vi "Logger.Variant.FindData4.vi"() -> ()   [LabVIEW 2016] (continued)
"976000107050008691717", "976000107050008701717", "976000107050008711717", "976000107050008721717", "976000107050008731717", "976000107050008741717", "976000107050008751717", "976000107050008761717", "976000107050008771717", "976000107050008781717", "976000107050008791717", "976000107050008801717", "976000107050008811717", "976000107050008821717", "976000107050008831717", "976000107050008841717", "976000107050008851717", "976000107050008861717", "976000107050008871717", "976000107050008881717", "976000107050008891717", "976000107050008901717", "976000107050008911717", "976000107050008921717", "976000107050008931717", "976000107050008941717", "976000107050008951717", "976000107050008961717", "976000107050008971717", "976000107050008981717", "976000107050008991717", "976000107050009001717", "976000107050009011717", "976000107050009021717", "976000107050009031717", "976000107050009041717", "976000107050009051717", "976000107050009061717", "976000107050009071717", "976000107050009081717", "976000107050009091717", "976000107050009101717", "976000107050009111717", "976000107050009121717", "976000107050009131717", "976000107050009141717", "976000107050009151717", "976000107050009161717", "976000107050009171717", "976000107050009181717", "976000107050009191717", "976000107050009201717", "976000107050009211717", "976000107050009221717", "976000107050009231717", "976000107050009241717", "976000107050009251717", "976000107050009261717", "976000107050009271717", "976000107050009281717", "976000107050009291717", "976000107050009301717", "976000107050009311717", "976000107050009321717", "976000107050009331717", "976000107050009341717", "976000107050009351717", "976000107050009361717", "976000107050009371717", "976000107050009381717", "976000107050009391717", "976000107050009401717", "976000107050009411717", "976000107050009421717", "976000107050009431717", "976000107050009441717", "976000107050009451717", "976000107050009461717", "976000107050009471717", "976000107050009481717", "976000107050009491717", "976000107050009501717", "976000107050009511717", "976000107050009521717", "976000107050009531717", "976000107050009541717", "976000107050009551717", "976000107050009561717", "976000107050009571717", "976000107050009581717", "976000107050009591717", "976000107050009601717", "976000107050009611717", "976000107050009621717", "976000107050009631717", "976000107050009641717", "976000107050009651717", "976000107050009661717", "976000107050009671717", "976000107050009681717", "976000107050009691717", "976000107050009701717", "976000107050009711717", "976000107050009721717", "976000107050009731717", "976000107050009741717", "976000107050009751717", "976000107050009761717", "976000107050009771717", "976000107050009781717", "976000107050009791717", "976000107050009801717", "976000107050009811717", "976000107050009821717"]}, {"Product"="4802040310", "Plate"="8990538144", "Path"=path "D:/Maszup/WABCO/SVN/LaserMarkingStation/SOFTWARE/logs/results2/new/170426104556 899 053 814 4.tdms", "Serials"=["480204031053243421717", "480204031053243431717", "480204031053243441717", "480204031053243451717", "480204031053243461717", "480204031053243471717", "480204031053243481717", "480204031053243491717", "480204031053243501717", "480204031053243511717", "480204031053243521717", "480204031053243531717", "480204031053243541717", "480204031053243551717", "480204031053243561717", "480204031053243571717", "480204031053243581717", "480204031053243591717", "480204031053243601717", "480204031053243611717", "480204031053243621717", "480204031053243631717", "480204031053243641717", "480204031053243651717", "480204031053243661717", "480204031053243671717", "480204031053243681717", "480204031053243691717", "480204031053243701717", "480204031053243711717", "480204031053243721717", "480204031053243731717", "480204031053243741717", "480204031053243751717", "480204031053243761717", "480204031053243771717", "480204031053243781717", "480204031053243791717", "480204031053243801717", "480204031053243811717", "480204031053243821717", "480204031053243831717", "480204031053243841717", "480204031053243851717", "480204031053243861717"]}, {"Product"="4728900600", "Plate"="8990538144", "Path"=path "D:/Maszup/WABCO/SVN/LaserMarkingStation/SOFTWARE/logs/results2/new/170426104959 899 053 814 4.tdms", "Serials"=["472890060053240011717", "472890060053240021717", "472890060053240031717", "472890060053240041717", "472890060053240051717", "472890060053240061717", "472890060053240071717", "472890060053240081717", "472890060053240091717", "472890060053240101717", "472890060053240111717", "472890060053240121717", "472890060053240131717", "472890060053240141717", "472890060053240151717", "472890060053240161717", "472890060053240171717", "472890060053240181717", "472890060053240191717", "472890060053240201717", "472890060053240211717", "472890060053240221717", "472890060053240231717", "472890060053240241717"]}, {"Product"="4728900600", "Plate"="8990538144", "Path"=path "D:/Maszup/WABCO/SVN/LaserMarkingStation/SOFTWARE/logs/results2/new/170426105319 899 053 814 4.tdms", "Serials"=["472890060053240251717", "472890060053240261717", "472890060053240271717", "472890060053240281717", "472890060053240291717", "472890060053240301717", "472890060053240311717", "472890060053240321717", "472890060053240331717", "472890060053240341717", "472890060053240351717", "472890060053240361717", "472890060053240371717", "472890060053240381717", "472890060053240391717", "472890060053240401717", "472890060053240411717", "472890060053240421717", "472890060053240431717", "472890060053240441717", "472890060053240451717", "472890060053240461717", "472890060053240471717", "472890060053240481717"]}, {"Product"="4801020650", "Plate"="8990538034", "Path"=path "D:/Maszup/WABCO/SVN/LaserMarkingStation/SOFTWARE/logs/results2/new/170426105704 899 053 803 4.tdms", "Serials"=["48010206500635291717", "48010206500635301717", "48010206500635311717", "48010206500635321717", "48010206500635331717", "48010206500635341717", "48010206500635351717", "48010206500635361717", "48010206500635371717", "48010206500635381717", "48010206500635391717", "48010206500635401717", "48010206500635411717", "48010206500635421717", "48010206500635431717", "48010206500635441717", "48010206500635451717", "48010206500635461717", "48010206500635471717", "48010206500635481717", "48010206500635491717", "48010206500635501717", "48010206500635511717", "48010206500635521717", "48010206500635531717", "48010206500635541717", "48010206500635551717", "48010206500635561717", "48010206500635571717", "48010206500635581717", "48010206500635591717", "48010206500635601717", "48010206500635611717", "48010206500635621717", "48010206500635631717", "48010206500635641717"]}, {"Product"="4801020650", "Plate"="8990538034", "Path"=path "D:/Maszup/WABCO/SVN/LaserMarkingStation/SOFTWARE/logs/results2/new/170426110126 899 053 803 4.tdms", "Serials"=["48010206500634931717", "48010206500634941717", "48010206500634951717", "48010206500634961717", "48010206500634971717", "48010206500634981717", "48010206500634991717", "48010206500635001717", "48010206500635011717", "48010206500635021717", "48010206500635031717", "48010206500635041717", "48010206500635051717", "48010206500635061717", "48010206500635071717", "48010206500635081717", "48010206500635091717", "48010206500635101717", "48010206500635111717", "48010206500635121717", "48010206500635131717", "48010206500635141717", "48010206500635151717", "48010206500635161717", "48010206500635171717", "48010206500635181717", "48010206500635191717", "48010206500635201717", "48010206500635211717", "48010206500635221717", "48010206500635231717", "48010206500635241717", "48010206500635251717", "48010206500635261717", "48010206500635271717", "48010206500635281717"]}, {"Product"="4801020630", "Plate"="8990538034", "Path"=path "D:/Maszup/WABCO/SVN/LaserMarkingStation/SOFTWARE/logs/results2/new/170426110834 899 053 803 4.tdms", "Serials"=["48010206303717401717", "48010206303717411717"]}, {"Product"="4801020630", "Plate"="8990538034", "Path"=path "D:/Maszup/WABCO/SVN/LaserMarkingStation/SOFTWARE/logs/results2/new/170426111204 899 053 803 4.tdms", "Serials"=["48010206303717401717", "48010206303717411717", "48010206303717421717", "48010206303717431717"]}, {"Product"="4801020630", "Plate"="8990538034", "Path"=path "D:/Maszup/WABCO/SVN/LaserMarkingStation/SOFTWARE/logs/results2/new/170426111329 899 053 803 4.tdms", "Serials"=["48010206303717401717", "48010206303717411717", "48010206303717421717", "48010206303717431717", "48010206303717441717", "48010206303717451717", "48010206303717461717", "48010206303717471717", "48010206303717481717", "48010206303717491717", "48010206303717501717", "48010206303717511717", "48010206303717521717", "48010206303717531717", "48010206303717541717", "48010206303717551717", "48010206303717561717", "48010206303717571717", "48010206303717581717", "48010206303717591717", "48010206303717601717", "48010206303717611717", "48010206303717621717", "48010206303717631717"]}, {"Product"="4801020630", "Plate"="8990538034", "Path"=path "D:/Maszup/WABCO/SVN/LaserMarkingStation/SOFTWARE/logs/results2/new/170426112001 899 053 803 4.tdms", "Serials"=["48010206303715961717", "48010206303715971717", "48010206303715981717", "48010206303715991717", "48010206303716001717", "48010206303716011717", "48010206303716021717", "48010206303716031717", "48010206303716041717", "48010206303716051717", "48010206303716061717", "48010206303716071717", "48010206303716081717", "48010206303716091717", "48010206303716101717", "48010206303716111717", "48010206303716121717", "48010206303716131717", "48010206303716141717", "48010206303716151717", "48010206303716161717", "48010206303716171717", "48010206303716181717", "48010206303716191717", "48010206303716201717", "48010206303716211717", "48010206303716221717", "48010206303716231717", "48010206303716241717", "48010206303716251717", "48010206303716261717", "48010206303716271717", "48010206303716281717", "48010206303716291717", "48010206303716301717", "48010206303716311717", "48010206303716321717", "48010206303716331717", "48010206303716341717", "48010206303716351717", "48010206303716361717", "48010206303716371717", "48010206303716381717", "48010206303716391717", "48010206303716401717", "48010206303716411717", "48010206303716421717", "48010206303716431717", "48010206303716441717", "48010206303716451717", "48010206303716461717", "48010206303716471717", "48010206303716481717", "48010206303716491717", "48010206303716501717", "48010206303716511717", "48010206303716521717", "48010206303716531717", "48010206303716541717", "48010206303716551717", "48010206303716561717", "48010206303716571717", "48010206303716581717", "48010206303716591717", "48010206303716601717", "48010206303716611717", "48010206303716621717", "48010206303716631717", "48010206303716641717", "48010206303716651717", "48010206303716661717", "48010206303716671717", "48010206303716681717", "48010206303716691717", "48010206303716701717", "48010206303716711717", "48010206303716721717", "48010206303716731717", "48010206303716741717", "48010206303716751717", "48010206303716761717", "48010206303716771717", "48010206303716781717", "48010206303716791717", "48010206303716801717", "48010206303716811717", "48010206303716821717", "48010206303716831717", "48010206303716841717", "48010206303716851717", "48010206303716861717", "48010206303716871717", "48010206303716881717", "48010206303716891717", "48010206303716901717", "48010206303716911717", "48010206303716921717", "48010206303716931717", "48010206303716941717", "48010206303716951717", "48010206303716961717", "48010206303716971717", "48010206303716981717", "48010206303716991717", "48010206303717001717", "48010206303717011717", "48010206303717021717", "48010206303717031717", "48010206303717041717", "48010206303717051717", "48010206303717061717", "48010206303717071717", "48010206303717081717", "48010206303717091717", "48010206303717101717", "48010206303717111717", "48010206303717121717", "48010206303717131717", "48010206303717141717", "48010206303717151717", "48010206303717161717", "48010206303717171717", "48010206303717181717", "48010206303717191717", "48010206303717201717", "48010206303717211717", "48010206303717221717", "48010206303717231717", "48010206303717241717", "48010206303717251717", "48010206303717261717", "48010206303717271717", "48010206303717281717", "48010206303717291717", "48010206303717301717", "48010206303717311717", "48010206303717321717", "48010206303717331717", "48010206303717341717", "48010206303717351717", "48010206303717361717", "48010206303717371717", "48010206303717381717", "48010206303717391717"]}, {"Product"="4728901120", "Plate"="8990538144", "Path"=path "D:/Maszup/WABCO/SVN/LaserMarkingStation/SOFTWARE/logs/results2/new/170426113518 899 053 814 4.tdms", "Serials"=["472890112055001041717", "472890112055001051717", "472890112055001061717", "472890112055001071717", "472890112055001081717", "472890112055001091717", "472890112055001101717", "472890112055001111717", "472890112055001121717", "472890112055001131717", "472890112055001141717", "472890112055001151717", "472890112055001161717", "472890112055001171717", "472890112055001181717", "472890112055001191717", "472890112055001201717", "472890112055001211717", "472890112055001221717", "472890112055001231717", "472890112055001241717", "472890112055001251717", "472890112055001261717", "472890112055001271717", "472890112055001281717", "472890112055001291717", "472890112055001301717", "472890112055001311717", "472890112055001321717", "472890112055001331717", "472890112055001341717", "472890112055001351717", "472890112055001361717", "472890112055001371717", "472890112055001381717", "472890112055001391717"]}, {"Product"="4729051110", "Plate"="8990538144", "Path"=path "D:/Maszup/WABCO/SVN/LaserMarkingStation/SOFTWARE/logs/results2/new/170426114140 899 053 814 4.tdms", "Serials"=["472905111065780911717", "472905111065780921717", "472905111065780931717", "472905111065780941717", "472905111065780951717", "472905111065780961717", "472905111065780971717", "472905111065780981717", "472905111065780991717", "472905111065781001717", "472905111065781011717", "472905111065781021717", "472905111065781031717", "472905111065781041717", "472905111065781051717", "472905111065781061717", "472905111065781071717", "472905111065781081717", "472905111065781091717", "472905111065781101717"]}, {"Product"="4800030470", "Plate"="8990538144", "Path"=path "D:/Maszup/WABCO/SVN/LaserMarkingStation/SOFTWARE/logs/results2/new/170426115616 899 053 814 4.tdms", "Serials"=["480003047053240031717", "480003047053240041717", "480003047053240051717", "480003047053240061717", "480003047053240071717", "480003047053240081717", "480003047053240091717", "480003047053240101717", "480003047053240111717", "480003047053240121717", "480003047053240131717", "480003047053240141717", "480003047053240151717", "480003047053240161717", "480003047053240171717", "480003047053240181717", "480003047053240191717", "480003047053240201717", "480003047053240211717", "480003047053240221717", "480003047053240231717", "480003047053240241717", "480003047053240251717", "480003047053240261717", "480003047053240271717", "480003047053240281717", "480003047053240291717", "480003047053240301717", "480003047053240311717", "480003047053240321717", "480003047053240331717", "480003047053240341717", "480003047053240351717", "480003047053240361717", "480003047053240371717", "480003047053240381717", "480003047053240391717", "480003047053240401717", "480003047053240411717", "480003047053240421717"]}, {"Product"="4640061000", "Plate"="8990538034", "Path"=path "D:/Maszup/WABCO/SVN/LaserMarkingStation/SOFTWARE/logs/results2/new/170426120944 899 053 803 4.tdms", "Serials"=["46400610000312521717", "46400610000312531717"]}, {"Product"="4800030470", "Plate"="8990538144", "Path"=path "D:/Maszup/WABCO/SVN/LaserMarkingStation/SOFTWARE/logs/results2/new/170426121217 899 053 814 4.tdms", "Serials"=["480003047053240431717", "480003047053240441717", "480003047053240451717", "480003047053240461717", "480003047053240471717", "480003047053240481717", "480003047053240491717", "480003047053240501717", "480003047053240511717", "480003047053240521717", "480003047053240531717", "480003047053240541717", "480003047053240551717", "480003047053240561717", "480003047053240571717", "480003047053240581717", "480003047053240591717", "480003047053240601717", "480003047053240611717", "480003047053240621717", "480003047053240631717", "480003047053240641717", "480003047053240651717", "480003047053240661717", "480003047053240671717", "480003047053240681717", "480003047053240691717", "480003047053240701717", "480003047053240711717", "480003047053240721717", "480003047053240731717", "480003047053240741717", "480003047053240751717", "480003047053240761717", "480003047053240771717", "480003047053240781717", "480003047053240791717", "480003047053240801717", "480003047053240811717", "480003047053240821717"]}, {"Product"="9650010530", "Plate"="8990538144", "Path"=path "D:/Maszup/WABCO/SVN/LaserMarkingStation/SOFTWARE/logs/results2/new/170426150118 899 053 814 4.tdms", "Serials"=["965001053000148491717", "965001053000148501717", "965001053000148511717", "965001053000148521717", "965001053000148531717", "965001053000148541717", "965001053000148551717", "965001053000148561717", "965001053000148571717", "965001053000148581717", "965001053000148591717", "965001053000148601717"]}, {"Product"="9650010530", "Plate"="8990538144", "Path"=path "D:/Maszup/WABCO/SVN/LaserMarkingStation/SOFTWARE/logs/results2/new/170426150640 899 053 814 4.tdms", "Serials"=["965001053000148611717", "965001053000148621717", "965001053000148631717", "965001053000148641717", "965001053000148651717", "965001053000148661717", "965001053000148671717", "965001053000148681717", "965001053000148691717", "965001053000148701717", "965001053000148711717", "965001053000148721717"]}, {"Product"="4800030600", "Plate"="8990501474", "Path"=path "D:/Maszup/WABCO/SVN/LaserMarkingStation/SOFTWARE/logs/results2/new/170426181430 899 050 147 4.tdms", "Serials"=["480003060053240011717", "480003060053240021717", "480003060053240031717", "480003060053240041717", "480003060053240051717", "480003060053240061717", "480003060053240071717", "480003060053240081717", "480003060053240091717", "480003060053240101717", "480003060053240111717", "480003060053240121717", "480003060053240131717", "480003060053240141717", "480003060053240151717", "480003060053240161717", "480003060053240171717", "480003060053240181717", "480003060053240191717", "480003060053240201717", "480003060053240211717", "480003060053240221717", "480003060053240231717", "480003060053240241717"]}, {"Product"="4800030600", "Plate"="8990501474", "Path"=path "D:/Maszup/WABCO/SVN/LaserMarkingStation/SOFTWARE/logs/results2/new/170426181931 899 050 147 4.tdms", "Serials"=["480003060053240251717", "480003060053240261717", "480003060053240271717", "480003060053240281717", "480003060053240291717", "480003060053240301717", "480003060053240311717", "480003060053240321717", "480003060053240331717", "480003060053240341717", "480003060053240351717", "480003060053240361717", "480003060053240371717", "480003060053240381717", "480003060053240391717", "480003060053240401717", "480003060053240411717", "480003060053240421717", "480003060053240431717", "480003060053240441717", "480003060053240451717", "480003060053240461717", "480003060053240471717", "480003060053240481717"]}, {"Product"="4800030500", "Plate"="8990501474", "Path"=path "D:/Maszup/WABCO/SVN/LaserMarkingStation/SOFTWARE/logs/results2/new/170426215055 899 050 147 4.tdms", "Serials"=["480003050053255101717", "480003050053255111717", "480003050053255121717", "480003050053255131717", "480003050053255141717", "480003050053255151717", "480003050053255161717", "480003050053255171717", "480003050053255181717", "480003050053255191717", "480003050053255201717", "480003050053255211717", "480003050053255221717", "480003050053255231717", "480003050053255241717", "480003050053255251717", "480003050053255261717", "480003050053255271717", "480003050053255281717", "480003050053255291717", "480003050053255301717", "480003050053255311717", "480003050053255321717", "480003050053255331717", "480003050053255341717", "480003050053255351717", "480003050053255361717", "480003050053255371717", "480003050053255381717", "480003050053255391717", "480003050053255401717", "480003050053255411717", "480003050053255421717", "480003050053255431717", "480003050053255441717", "480003050053255451717", "480003050053255461717", "480003050053255471717", "480003050053255481717", "480003050053255491717", "480003050053255501717", "480003050053255511717", "480003050053255521717", "480003050053255531717", "480003050053255541717", "480003050053255551717", "480003050053255561717", "480003050053255571717", "480003050053255581717", "480003050053255591717", "480003050053255601717", "480003050053255611717", "480003050053255621717", "480003050053255631717", "480003050053255641717", "480003050053255651717", "480003050053255661717", "480003050053255671717", "480003050053255681717", "480003050053255691717", "480003050053255701717", "480003050053255711717", "480003050053255721717", "480003050053255731717", "480003050053255741717", "480003050053255751717", "480003050053255761717", "480003050053255771717", "480003050053255781717", "480003050053255791717", "480003050053255801717", "480003050053255811717", "480003050053255821717", "480003050053255831717", "480003050053255841717", "480003050053255851717", "480003050053255861717", "480003050053255871717", "480003050053255881717", "480003050053255891717", "480003050053255901717", "480003050053255911717", "480003050053255921717", "480003050053255931717", "480003050053255941717", "480003050053255951717", "480003050053255961717", "480003050053255971717", "480003050053255981717", "480003050053255991717", "480003050053256001717", "480003050053256011717", "480003050053256021717", "480003050053256031717", "480003050053256041717", "480003050053256051717", "480003050053256061717", "480003050053256071717", "480003050053256081717", "480003050053256091717", "480003050053256101717", "480003050053256111717", "480003050053256121717", "480003050053256131717", "480003050053256141717", "480003050053256151717", "480003050053256161717", "480003050053256171717", "480003050053256181717", "480003050053256191717", "480003050053256201717", "480003050053256211717", "480003050053256221717", "480003050053256231717", "480003050053256241717", "480003050053256251717", "480003050053256261717", "480003050053256271717", "480003050053256281717", "480003050053256291717", "480003050053256301717", "480003050053256311717", "480003050053256321717", "480003050053256331717", "480003050053256341717", "480003050053256351717", "480003050053256361717", "480003050053256371717", "480003050053256381717", "480003050053256391717", "480003050053256401717", "480003050053256411717", "480003050053256421717", "480003050053256431717", "480003050053256441717", "480003050053256451717", "480003050053256461717", "480003050053256471717", "480003050053256481717", "480003050053256491717", "480003050053256501717", "480003050053256511717", "480003050053256521717", "480003050053256531717", "480003050053256541717", "480003050053256551717", "480003050053256561717", "480003050053256571717", "480003050053256581717", "480003050053256591717", "480003050053256601717", "480003050053256611717", "480003050053256621717", "480003050053256631717", "480003050053256641717", "480003050053256651717", "480003050053256661717", "480003050053256671717", "480003050053256681717", "480003050053256691717", "480003050053256701717", "480003050053256711717", "480003050053256721717", "480003050053256731717", "480003050053256741717", "480003050053256751717", "480003050053256761717", "480003050053256771717", "480003050053256781717", "480003050053256791717", "480003050053256801717", "480003050053256811717", "480003050053256821717", "480003050053256831717", "480003050053256841717", "480003050053256851717", "480003050053256861717", "480003050053256871717", "480003050053256881717", "480003050053256891717", "480003050053256901717", "480003050053256911717", "480003050053256921717", "480003050053256931717", "480003050053256941717", "480003050053256951717", "480003050053256961717", "480003050053256971717", "480003050053256981717", "480003050053256991717", "480003050053257001717", "480003050053257011717"]}, {"Product"="4728800010", "Plate"="8990538154", "Path"=path "D:/Maszup/WABCO/SVN/LaserMarkingStation/SOFTWARE/logs/results2/new/170427002818 899 053 815 4.tdms", "Serials"=["472880001053240011717"]}, {"Product"="9760001010", "Plate"="8990501474", "Path"=path "D:/Maszup/WABCO/SVN/LaserMarkingStation/SOFTWARE/logs/results2/new/170427061903 899 050 147 4.tdms", "Serials"=["976000101050001241717", "976000101050001251717", "976000101050001261717", "976000101050001271717", "976000101050001281717", "976000101050001291717", "976000101050001301717", "976000101050001311717", "976000101050001321717", "976000101050001331717", "976000101050001341717", "976000101050001351717", "976000101050001361717", "976000101050001371717", "976000101050001381717", "976000101050001391717", "976000101050001401717", "976000101050001411717", "976000101050001421717", "976000101050001431717", "976000101050001441717", "976000101050001451717", "976000101050001461717", "976000101050001471717", "976000101050001481717", "976000101050001491717", "976000101050001501717", "976000101050001511717", "976000101050001521717", "976000101050001531717", "976000101050001541717", "976000101050001551717", "976000101050001561717", "976000101050001571717", "976000101050001581717", "976000101050001591717", "976000101050001601717", "976000101050001611717", "976000101050001621717", "976000101050001631717", "976000101050001641717", "976000101050001651717", "976000101050001661717", "976000101050001671717", "976000101050001681717", "976000101050001691717", "976000101050001701717", "976000101050001711717"]}, {"Product"="4640060027", "Plate"="8990502914", "Path"=path "D:/Maszup/WABCO/SVN/LaserMarkingStation/SOFTWARE/logs/results2/new/170427093837 899 050 291 4.tdms", "Serials"=["46400600270139471717", "46400600270139481717", "46400600270139491717", "46400600270139501717", "46400600270139511717", "46400600270139521717", "46400600270139531717", "46400600270139541717", "46400600270139551717", "46400600270139561717", "46400600270139571717", "46400600270139581717", "46400600270139591717", "46400600270139601717", "46400600270139611717", "46400600270139621717", "46400600270139631717", "46400600270139641717", "46400600270139651717", "46400600270139661717", "46400600270139671717", "46400600270139681717", "46400600270139691717", "46400600270139701717", "46400600270139711717", "46400600270139721717", "46400600270139731717", "46400600270139741717", "46400600270139751717", "46400600270139761717", "46400600270139771717", "46400600270139781717", "46400600270139791717", "46400600270139801717", "46400600270139811717", "46400600270139821717", "46400600270139831717", "46400600270139841717", "46400600270139851717", "46400600270139861717", "46400600270139871717", "46400600270139881717", "46400600270139891717", "46400600270139901717", "46400600270139911717", "46400600270139921717", "46400600270139931717", "46400600270139941717", "46400600270139951717", "46400600270139961717", "46400600270139971717", "46400600270139981717", "46400600270139991717"]}, {"Product"="8840494120", "Plate"="8990538144", "Path"=path "D:/Maszup/WABCO/SVN/LaserMarkingStation/SOFTWARE/logs/results2/new/170427124622 899 053 814 4.tdms", "Serials"=["884049412000000161717", "884049412000000171717", "884049412000000181717"]}, {"Product"="4800030500", "Plate"="8990501474", "Path"=path "D:/Maszup/WABCO/SVN/LaserMarkingStation/SOFTWARE/logs/results2/new/170427130233 899 050 147 4.tdms", "Serials"=["480003050053257021717", "480003050053257031717", "480003050053257041717", "480003050053257051717", "480003050053257061717", "480003050053257071717", "480003050053257081717", "480003050053257091717", "480003050053257101717", "480003050053257111717", "480003050053257121717", "480003050053257131717", "480003050053257141717", "480003050053257151717", "480003050053257161717", "480003050053257171717", "480003050053257181717", "480003050053257191717", "480003050053257201717", "480003050053257211717", "480003050053257221717", "480003050053257231717", "480003050053257241717", "480003050053257251717", "480003050053257261717", "480003050053257271717", "480003050053257281717", "480003050053257291717", "480003050053257301717", "480003050053257311717", "480003050053257321717", "480003050053257331717", "480003050053257341717", "480003050053257351717", "480003050053257361717", "480003050053257371717", "480003050053257381717", "480003050053257391717", "480003050053257401717", "480003050053257411717", "480003050053257421717", "480003050053257431717", "480003050053257441717", "480003050053257451717", "480003050053257461717", "480003050053257471717", "480003050053257481717", "480003050053257491717", "480003050053257501717", "480003050053257511717", "480003050053257521717", "480003050053257531717", "480003050053257541717", "480003050053257551717", "480003050053257561717", "480003050053257571717", "480003050053257581717", "480003050053257591717", "480003050053257601717", "480003050053257611717", "480003050053257621717", "480003050053257631717", "480003050053257641717", "480003050053257651717"]}, {"Product"="4800030500", "Plate"="8990501474", "Path"=path "D:/Maszup/WABCO/SVN/LaserMarkingStation/SOFTWARE/logs/results2/new/170427190006 899 050 147 4.tdms", "Serials"=["480003050053257661717", "480003050053257671717", "480003050053257681717", "480003050053257691717", "480003050053257701717", "480003050053257711717", "480003050053257721717", "480003050053257731717", "480003050053257741717", "480003050053257751717", "480003050053257761717", "480003050053257771717", "480003050053257781717", "480003050053257791717", "480003050053257801717", "480003050053257811717", "480003050053257821717", "480003050053257831717", "480003050053257841717", "480003050053257851717", "480003050053257861717", "480003050053257871717", "480003050053257881717", "480003050053257891717", "480003050053257901717", "480003050053257911717", "480003050053257921717", "480003050053257931717", "480003050053257941717", "480003050053257951717", "480003050053257961717", "480003050053257971717", "480003050053257981717", "480003050053257991717", "480003050053258001717", "480003050053258011717", "480003050053258021717", "480003050053258031717", "480003050053258041717", "480003050053258051717", "480003050053258061717", "480003050053258071717", "480003050053258081717", "480003050053258091717", "480003050053258101717", "480003050053258111717", "480003050053258121717", "480003050053258131717", "480003050053258141717", "480003050053258151717", "480003050053258161717", "480003050053258171717", "480003050053258181717", "480003050053258191717", "480003050053258201717", "480003050053258211717", "480003050053258221717", "480003050053258231717", "480003050053258241717", "480003050053258251717", "480003050053258261717", "480003050053258271717", "480003050053258281717", "480003050053258291717", "480003050053258301717", "480003050053258311717", "480003050053258321717", "480003050053258331717", "480003050053258341717", "480003050053258351717", "480003050053258361717", "480003050053258371717", "480003050053258381717", "480003050053258391717", "480003050053258401717", "480003050053258411717", "480003050053258421717", "480003050053258431717", "480003050053258441717", "480003050053258451717", "480003050053258461717", "480003050053258471717", "480003050053258481717", "480003050053258491717", "480003050053258501717", "480003050053258511717", "480003050053258521717", "480003050053258531717", "480003050053258541717", "480003050053258551717", "480003050053258561717", "480003050053258571717", "480003050053258581717", "480003050053258591717", "480003050053258601717", "480003050053258611717", "480003050053258621717", "480003050053258631717", "480003050053258641717", "480003050053258651717", "480003050053258661717", "480003050053258671717", "480003050053258681717", "480003050053258691717", "480003050053258701717", "480003050053258711717", "480003050053258721717", "480003050053258731717", "480003050053258741717", "480003050053258751717", "480003050053258761717", "480003050053258771717", "480003050053258781717", "480003050053258791717", "480003050053258801717", "480003050053258811717", "480003050053258821717", "480003050053258831717", "480003050053258841717", "480003050053258851717", "480003050053258861717", "480003050053258871717", "480003050053258881717", "480003050053258891717", "480003050053258901717", "480003050053258911717", "480003050053258921717", "480003050053258931717", "480003050053258941717", "480003050053258951717", "480003050053258961717", "480003050053258971717", "480003050053258981717", "480003050053258991717", "480003050053259001717", "480003050053259011717", "480003050053259021717", "480003050053259031717", "480003050053259041717", "480003050053259051717", "480003050053259061717", "480003050053259071717", "480003050053259081717", "480003050053259091717", "480003050053259101717", "480003050053259111717", "480003050053259121717", "480003050053259131717", "480003050053259141717", "480003050053259151717", "480003050053259161717", "480003050053259171717", "480003050053259181717", "480003050053259191717", "480003050053259201717", "480003050053259211717", "480003050053259221717", "480003050053259231717", "480003050053259241717", "480003050053259251717", "480003050053259261717", "480003050053259271717", "480003050053259281717", "480003050053259291717", "480003050053259301717", "480003050053259311717", "480003050053259321717", "480003050053259331717", "480003050053259341717", "480003050053259351717", "480003050053259361717", "480003050053259371717", "480003050053259381717", "480003050053259391717", "480003050053259401717", "480003050053259411717", "480003050053259421717", "480003050053259431717", "480003050053259441717", "480003050053259451717", "480003050053259461717", "480003050053259471717", "480003050053259481717", "480003050053259491717", "480003050053259501717", "480003050053259511717", "480003050053259521717", "480003050053259531717", "480003050053259541717", "480003050053259551717", "480003050053259561717", "480003050053259571717"]}, {"Product"="4800030500", "Plate"="8990501474", "Path"=path "D:/Maszup/WABCO/SVN/LaserMarkingStation/SOFTWARE/logs/results2/new/170427192330 899 050 147 4.tdms", "Serials"=["480003050053259581717", "480003050053259591717", "480003050053259601717", "480003050053259611717", "480003050053259621717", "480003050053259631717", "480003050053259641717", "480003050053259651717", "480003050053259661717", "480003050053259671717", "480003050053259681717", "480003050053259691717", "480003050053259701717", "480003050053259711717", "480003050053259721717", "480003050053259731717", "480003050053259741717", "480003050053259751717", "480003050053259761717", "480003050053259771717", "480003050053259781717", "480003050053259791717", "480003050053259801717", "480003050053259811717", "480003050053259821717", "480003050053259831717", "480003050053259841717", "480003050053259851717", "480003050053259861717", "480003050053259871717", "480003050053259881717", "480003050053259891717", "480003050053259901717", "480003050053259911717", "480003050053259921717", "480003050053259931717", "480003050053259941717", "480003050053259951717", "480003050053259961717", "480003050053259971717", "480003050053259981717", "480003050053259991717", "480003050053260001717", "480003050053260011717", "480003050053260021717", "480003050053260031717", "480003050053260041717", "480003050053260051717", "480003050053260061717", "480003050053260071717", "480003050053260081717", "480003050053260091717", "480003050053260101717", "480003050053260111717", "480003050053260121717", "480003050053260131717", "480003050053260141717", "480003050053260151717", "480003050053260161717", "480003050053260171717", "480003050053260181717", "480003050053260191717", "480003050053260201717", "480003050053260211717", "480003050053260221717", "480003050053260231717", "480003050053260241717", "480003050053260251717", "480003050053260261717", "480003050053260271717", "480003050053260281717", "480003050053260291717", "480003050053260301717", "480003050053260311717", "480003050053260321717", "480003050053260331717", "480003050053260341717", "480003050053260351717", "480003050053260361717", "480003050053260371717", "480003050053260381717", "480003050053260391717", "480003050053260401717", "480003050053260411717", "480003050053260421717", "480003050053260431717", "480003050053260441717", "480003050053260451717", "480003050053260461717", "480003050053260471717", "480003050053260481717", "480003050053260491717", "480003050053260501717", "480003050053260511717", "480003050053260521717", "480003050053260531717", "480003050053260541717", "480003050053260551717", "480003050053260561717", "480003050053260571717", "480003050053260581717", "480003050053260591717", "480003050053260601717", "480003050053260611717", "480003050053260621717", "480003050053260631717", "480003050053260641717", "480003050053260651717", "480003050053260661717", "480003050053260671717", "480003050053260681717", "480003050053260691717", "480003050053260701717", "480003050053260711717", "480003050053260721717", "480003050053260731717", "480003050053260741717", "480003050053260751717", "480003050053260761717", "480003050053260771717", "480003050053260781717", "480003050053260791717", "480003050053260801717", "480003050053260811717", "480003050053260821717", "480003050053260831717", "480003050053260841717", "480003050053260851717", "480003050053260861717", "480003050053260871717", "480003050053260881717", "480003050053260891717", "480003050053260901717", "480003050053260911717", "480003050053260921717", "480003050053260931717", "480003050053260941717", "480003050053260951717", "480003050053260961717", "480003050053260971717", "480003050053260981717", "480003050053260991717", "480003050053261001717", "480003050053261011717", "480003050053261021717", "480003050053261031717", "480003050053261041717", "480003050053261051717", "480003050053261061717", "480003050053261071717", "480003050053261081717", "480003050053261091717", "480003050053261101717", "480003050053261111717", "480003050053261121717", "480003050053261131717", "480003050053261141717", "480003050053261151717", "480003050053261161717", "480003050053261171717", "480003050053261181717", "480003050053261191717", "480003050053261201717", "480003050053261211717", "480003050053261221717", "480003050053261231717", "480003050053261241717", "480003050053261251717", "480003050053261261717", "480003050053261271717", "480003050053261281717", "480003050053261291717", "480003050053261301717", "480003050053261311717", "480003050053261321717", "480003050053261331717", "480003050053261341717", "480003050053261351717", "480003050053261361717", "480003050053261371717", "480003050053261381717", "480003050053261391717", "480003050053261401717", "480003050053261411717", "480003050053261421717", "480003050053261431717", "480003050053261441717", "480003050053261451717", "480003050053261461717", "480003050053261471717", "480003050053261481717", "480003050053261491717"]}, {"Product"="9760001070", "Plate"="8990538144", "Path"=path "D:/Maszup/WABCO/SVN/LaserMarkingStation/SOFTWARE/logs/results2/new/170427233224 899 053 814 4.tdms", "Serials"=["976000107050009831717", "976000107050009841717", "976000107050009851717", "976000107050009861717", "976000107050009871717"]}, {"Product"="9760001010", "Plate"="8990501474", "Path"=path "D:/Maszup/WABCO/SVN/LaserMarkingStation/SOFTWARE/logs/results2/new/170427233422 899 050 147 4.tdms", "Serials"=["976000101050001721717", "976000101050001731717", "976000101050001741717", "976000101050001751717", "976000101050001761717", "976000101050001771717", "976000101050001781717", "976000101050001791717", "976000101050001801717", "976000101050001811717", "976000101050001821717", "976000101050001831717", "976000101050001841717", "976000101050001851717", "976000101050001861717", "976000101050001871717", "976000101050001881717", "976000101050001891717", "976000101050001901717", "976000101050001911717", "976000101050001921717", "976000101050001931717", "976000101050001941717", "976000101050001951717", "976000101050001961717", "976000101050001971717", "976000101050001981717", "976000101050001991717", "976000101050002001717", "976000101050002011717", "976000101050002021717", "976000101050002031717", "976000101050002041717", "976000101050002051717", "976000101050002061717", "976000101050002071717", "976000101050002081717", "976000101050002091717", "976000101050002101717", "976000101050002111717", "976000101050002121717", "976000101050002131717", "976000101050002141717", "976000101050002151717", "976000101050002161717", "976000101050002171717", "976000101050002181717", "976000101050002191717"]}, {"Product"="9760001000", "Plate"="8990501474", "Path"=path "D:/Maszup/WABCO/SVN/LaserMarkingStation/SOFTWARE/logs/results2/new/170427234049 899 050 147 4.tdms", "Serials"=["976000100050000551717", "976000100050000561717"]}, {"Product"="8840550640", "Plate"="8990538144", "Path"=path "D:/Maszup/WABCO/SVN/LaserMarkingStation/SOFTWARE/logs/results2/new/170428092516 899 053 814 4.tdms", "Serials"=["884055064000000011717", "884055064000000021717", "884055064000000031717", "884055064000000041717", "884055064000000051717", "884055064000000061717", "884055064000000071717", "884055064000000081717", "884055064000000091717", "884055064000000101717", "884055064000000111717", "884055064000000121717", "884055064000000131717", "884055064000000141717", "884055064000000151717", "884055064000000161717"]}, {"Product"="8840475770", "Plate"="8990538144", "Path"=path "D:/Maszup/WABCO/SVN/LaserMarkingStation/SOFTWARE/logs/results2/new/170428111110 899 053 814 4.tdms", "Serials"=["884047577050000011717", "884047577050000021717"]}, {"Product"="8840437270", "Plate"="8990538144", "Path"=path "D:/Maszup/WABCO/SVN/LaserMarkingStation/SOFTWARE/logs/results2/new/170428111301 899 053 814 4.tdms", "Serials"=["884043727050000661717", "884043727050000671717", "884043727050000681717", "884043727050000691717", "884043727050000701717", "884043727050000711717", "884043727050000721717"]}, {"Product"="9650010550", "Plate"="8990538144", "Path"=path "D:/Maszup/WABCO/SVN/LaserMarkingStation/SOFTWARE/logs/results2/new/170428113602 899 053 814 4.tdms", "Serials"=["965001055001230191717", "965001055001230201717", "965001055001230211717", "965001055001230221717", "965001055001230231717", "965001055001230241717", "965001055001230251717", "965001055001230261717", "965001055001230271717", "965001055001230281717", "965001055001230291717", "965001055001230301717"]}, {"Product"="9650010550", "Plate"="8990538144", "Path"=path "D:/Maszup/WABCO/SVN/LaserMarkingStation/SOFTWARE/logs/results2/new/170428113814 899 053 814 4.tdms", "Serials"=["965001055001230311717", "965001055001230321717", "965001055001230331717", "965001055001230341717", "965001055001230351717", "965001055001230361717", "965001055001230371717", "965001055001230381717", "965001055001230391717", "965001055001230401717", "965001055001230411717", "965001055001230421717"]}, {"Product"="9650010550", "Plate"="8990538144", "Path"=path "D:/Maszup/WABCO/SVN/LaserMarkingStation/SOFTWARE/logs/results2/new/170428114248 899 053 814 4.tdms", "Serials"=["965001055001230431717", "965001055001230441717", "965001055001230451717", "965001055001230461717", "965001055001230471717", "965001055001230481717", "965001055001230491717", "965001055001230501717", "965001055001230511717", "965001055001230521717", "965001055001230531717", "965001055001230541717"]}, {"Product"="9650010550", "Plate"="8990538144", "Path"=path "D:/Maszup/WABCO/SVN/LaserMarkingStation/SOFTWARE/logs/results2/new/170428114529 899 053 814 4.tdms", "Serials"=["965001055001230551717", "965001055001230561717", "965001055001230571717", "965001055001230581717", "965001055001230591717", "965001055001230601717", "965001055001230611717", "965001055001230621717", "965001055001230631717", "965001055001230641717", "965001055001230651717", "965001055001230661717"]}, {"Product"="4800030580", "Plate"="8990501474", "Path"=path "D:/Maszup/WABCO/SVN/LaserMarkingStation/SOFTWARE/logs/results2/new/170428152705 899 050 147 4.tdms", "Serials"=["480003058053240671717", "480003058053240681717", "480003058053240691717", "480003058053240701717", "480003058053240711717", "480003058053240721717", "480003058053240731717", "480003058053240741717", "480003058053240751717", "480003058053240761717", "480003058053240771717", "480003058053240781717", "480003058053240791717", "480003058053240801717", "480003058053240811717", "480003058053240821717", "480003058053240831717", "480003058053240841717", "480003058053240851717", "480003058053240861717", "480003058053240871717", "480003058053240881717", "480003058053240891717", "480003058053240901717", "480003058053240911717", "480003058053240921717", "480003058053240931717", "480003058053240941717", "480003058053240951717", "480003058053240961717", "480003058053240971717", "480003058053240981717", "480003058053240991717", "480003058053241001717", "480003058053241011717", "480003058053241021717", "480003058053241031717", "480003058053241041717", "480003058053241051717", "480003058053241061717", "480003058053241071717", "480003058053241081717", "480003058053241091717", "480003058053241101717", "480003058053241111717", "480003058053241121717", "480003058053241131717", "480003058053241141717", "480003058053241151717", "480003058053241161717", "480003058053241171717", "480003058053241181717", "480003058053241191717", "480003058053241201717", "480003058053241211717", "480003058053241221717", "480003058053241231717", "480003058053241241717", "480003058053241251717", "480003058053241261717", "480003058053241271717", "480003058053241281717", "480003058053241291717", "480003058053241301717", "480003058053241311717", "480003058053241321717", "480003058053241331717", "480003058053241341717", "480003058053241351717", "480003058053241361717", "480003058053241371717", "480003058053241381717", "480003058053241391717", "480003058053241401717", "480003058053241411717", "480003058053241421717", "480003058053241431717", "480003058053241441717", "480003058053241451717", "480003058053241461717", "480003058053241471717", "480003058053241481717", "480003058053241491717", "480003058053241501717", "480003058053241511717", "480003058053241521717", "480003058053241531717", "480003058053241541717", "480003058053241551717", "480003058053241561717", "480003058053241571717", "480003058053241581717", "480003058053241591717", "480003058053241601717", "480003058053241611717", "480003058053241621717", "480003058053241631717", "480003058053241641717", "480003058053241651717", "480003058053241661717", "480003058053241671717", "480003058053241681717", "480003058053241691717", "480003058053241701717", "480003058053241711717", "480003058053241721717", "480003058053241731717", "480003058053241741717", "480003058053241751717", "480003058053241761717", "480003058053241771717", "480003058053241781717", "480003058053241791717", "480003058053241801717", "480003058053241811717", "480003058053241821717", "480003058053241831717", "480003058053241841717", "480003058053241851717", "480003058053241861717", "480003058053241871717", "480003058053241881717", "480003058053241891717", "480003058053241901717", "480003058053241911717", "480003058053241921717", "480003058053241931717", "480003058053241941717"]}, {"Product"="9760001000", "Plate"="8990501474", "Path"=path "D:/Maszup/WABCO/SVN/LaserMarkingStation/SOFTWARE/logs/results2/new/170428153838 899 050 147 4.tdms", "Serials"=["976000100050000571717", "976000100050000581717", "976000100050000591717", "976000100050000601717", "976000100050000611717", "976000100050000621717", "976000100050000631717", "976000100050000641717", "976000100050000651717", "976000100050000661717", "976000100050000671717", "976000100050000681717", "976000100050000691717", "976000100050000701717", "976000100050000711717", "976000100050000721717"]}, {"Product"="4800030500", "Plate"="8990501474", "Path"=path "D:/Maszup/WABCO/SVN/LaserMarkingStation/SOFTWARE/logs/results2/new/170428171435 899 050 147 4.tdms", "Serials"=["480003050053261501717", "480003050053261511717", "480003050053261521717", "480003050053261531717", "480003050053261541717", "480003050053261551717", "480003050053261561717", "480003050053261571717", "480003050053261581717", "480003050053261591717", "480003050053261601717", "480003050053261611717", "480003050053261621717", "480003050053261631717", "480003050053261641717", "480003050053261651717", "480003050053261661717", "480003050053261671717", "480003050053261681717", "480003050053261691717", "480003050053261701717", "480003050053261711717", "480003050053261721717", "480003050053261731717", "480003050053261741717", "480003050053261751717", "480003050053261761717", "480003050053261771717", "480003050053261781717", "480003050053261791717", "480003050053261801717", "480003050053261811717", "480003050053261821717", "480003050053261831717", "480003050053261841717", "480003050053261851717", "480003050053261861717", "480003050053261871717", "480003050053261881717", "480003050053261891717", "480003050053261901717", "480003050053261911717", "480003050053261921717", "480003050053261931717", "480003050053261941717", "480003050053261951717", "480003050053261961717", "480003050053261971717", "480003050053261981717", "480003050053261991717", "480003050053262001717", "480003050053262011717"]}, {"Product"="4640060027", "Plate"="8990502914", "Path"=path "D:/Maszup/WABCO/SVN/LaserMarkingStation/SOFTWARE/logs/results2/new/170428180206 899 050 291 4.tdms", "Serials"=["46400600270142401717", "46400600270142411717", "46400600270142421717", "46400600270142431717", "46400600270142441717", "46400600270142451717", "46400600270142461717", "46400600270142471717", "46400600270142481717", "46400600270142491717", "46400600270142501717", "46400600270142511717", "46400600270142521717", "46400600270142531717", "46400600270142541717", "46400600270142551717", "46400600270142561717", "46400600270142571717", "46400600270142581717", "46400600270142591717", "46400600270142601717", "46400600270142611717", "46400600270142621717", "46400600270142631717", "46400600270142641717", "46400600270142651717", "46400600270142661717", "46400600270142671717", "46400600270142681717", "46400600270142691717", "46400600270142701717", "46400600270142711717", "46400600270142721717", "46400600270142731717", "46400600270142741717", "46400600270142751717", "46400600270142761717", "46400600270142771717", "46400600270142781717", "46400600270142791717", "46400600270142801717", "46400600270142811717", "46400600270142821717", "46400600270142831717", "46400600270142841717", "46400600270142851717", "46400600270142861717", "46400600270142871717", "46400600270142881717", "46400600270142891717", "46400600270142901717", "46400600270142911717", "46400600270142921717", "46400600270142931717", "46400600270142941717", "46400600270142951717", "46400600270142961717", "46400600270142971717", "46400600270142981717", "46400600270142991717", "46400600270143001717", "46400600270143011717", "46400600270143021717", "46400600270143031717", "46400600270143041717", "46400600270143051717", "46400600270143061717", "46400600270143071717", "46400600270143081717", "46400600270143091717", "46400600270143101717", "46400600270143111717", "46400600270143121717", "46400600270143131717", "46400600270143141717", "46400600270143151717", "46400600270143161717", "46400600270143171717", "46400600270143181717", "46400600270143191717"]}, {"Product"="4728800010", "Plate"="8990538154", "Path"=path "D:/Maszup/WABCO/SVN/LaserMarkingStation/SOFTWARE/logs/results2/old/170420083829 899 053 815 4.tdms", "Serials"=["472880001050001511617", "472880001050001521617", "472880001050001531617", "472880001050001541617", "472880001050001551617", "472880001050001561617", "472880001050001571617", "472880001050001581617", "472880001050001591617", "472880001050001601617", "472880001050001611617", "472880001050001621617", "472880001050001631617", "472880001050001641617", "472880001050001651617"]}, {"Product"="9762001000", "Plate"="8990538144", "Path"=path "D:/Maszup/WABCO/SVN/LaserMarkingStation/SOFTWARE/logs/results2/old/170420085232 899 053 814 4.tdms", "Serials"=["976200100000003891617", "976200100000003901617", "976200100000003911617", "976200100000003921617", "976200100000003931617", "976200100000003941617", "976200100000003951617", "976200100000003961617"]}]
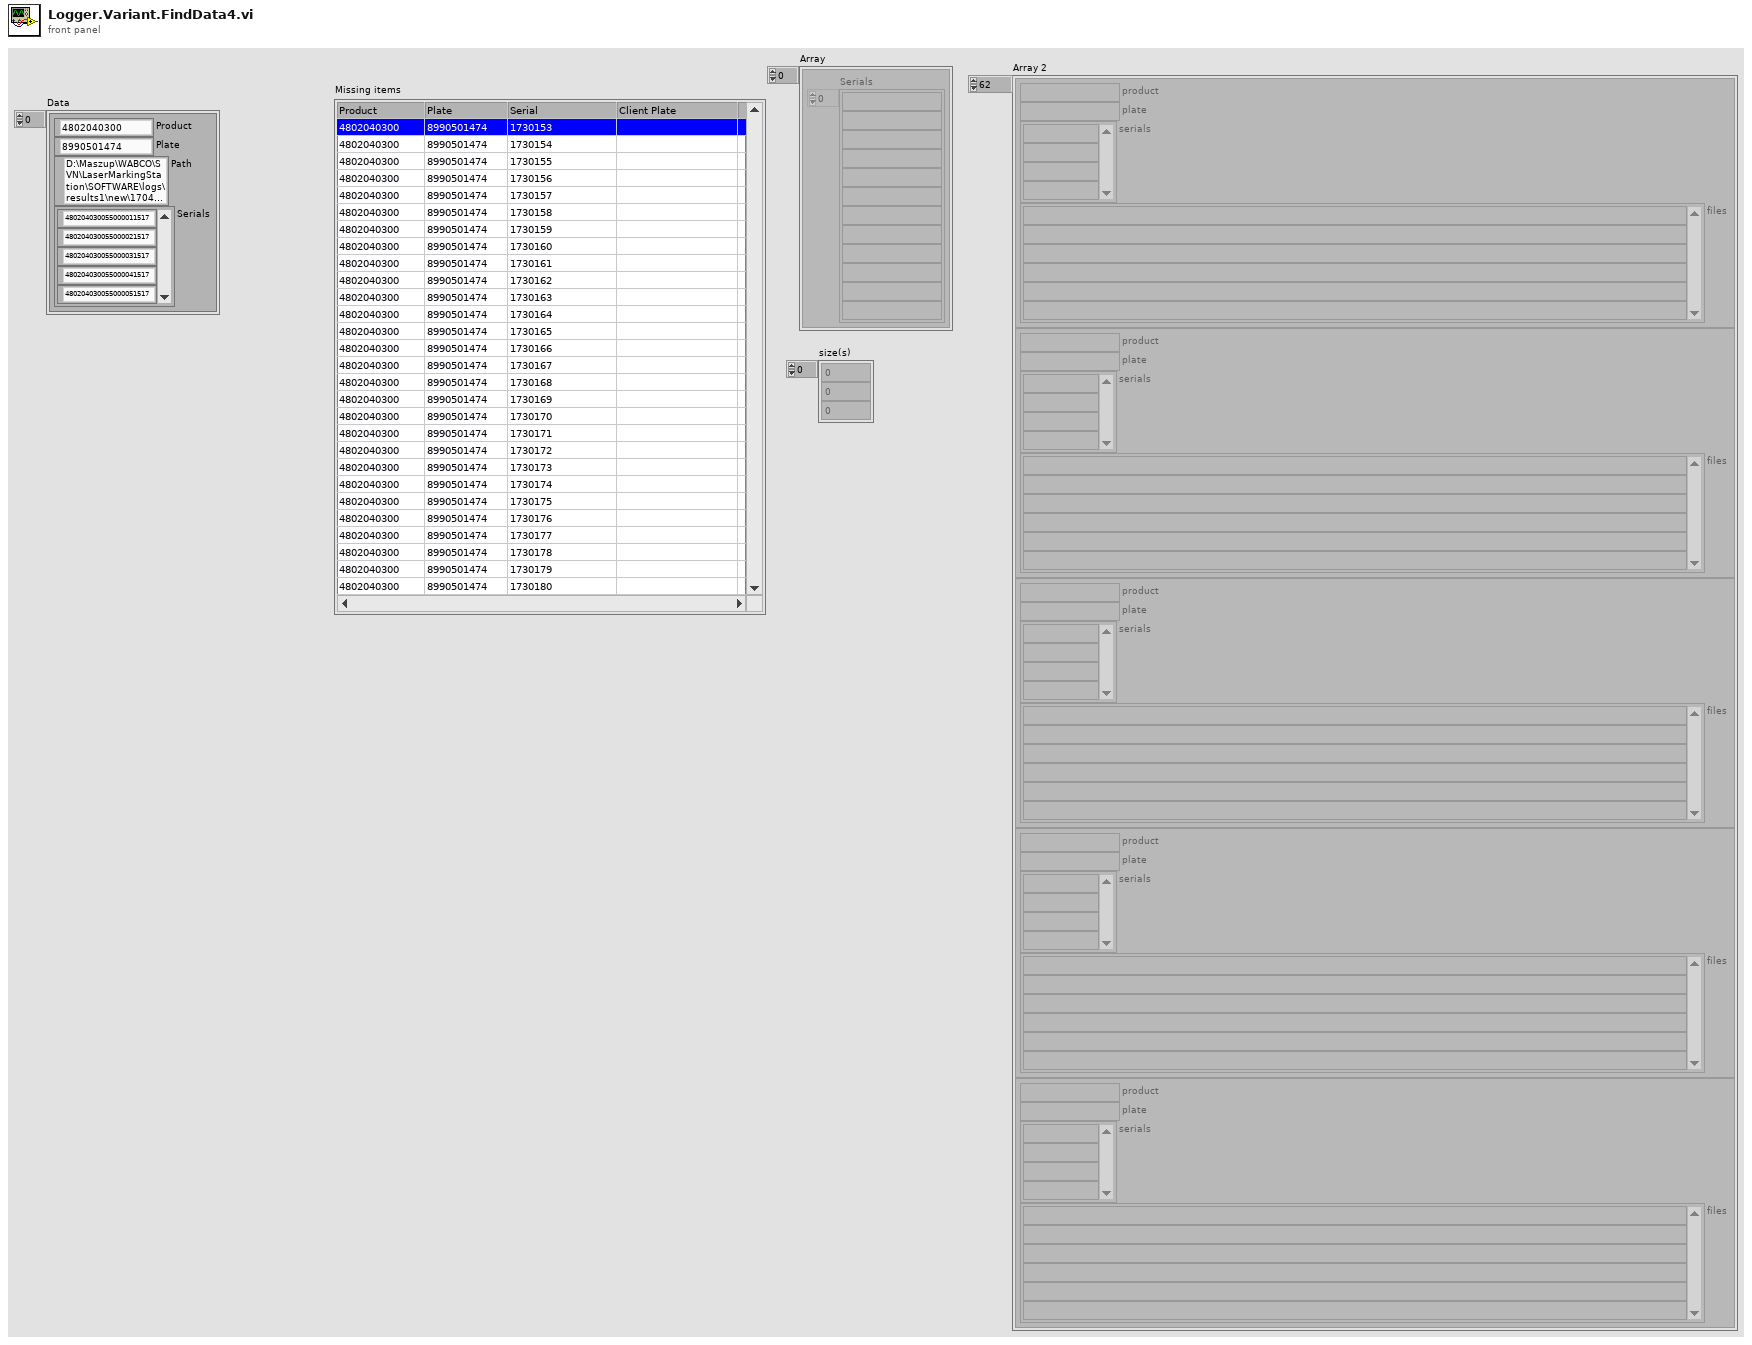
[diagram p1: front panel]
types:
  T1 = cluster{"product":string, "plate":string, "serials":string[], "files":string[]}[]
  T2 = cluster{"Product":string, "Plate":string, "Path":path, "Serials":string[]}[]
  T3 = cluster{"Product":string, "Plate":string, "Path":path, "Serials":string[]}
  T4 = cluster{"value":string, "value":string, string[], "unique values":string[]}
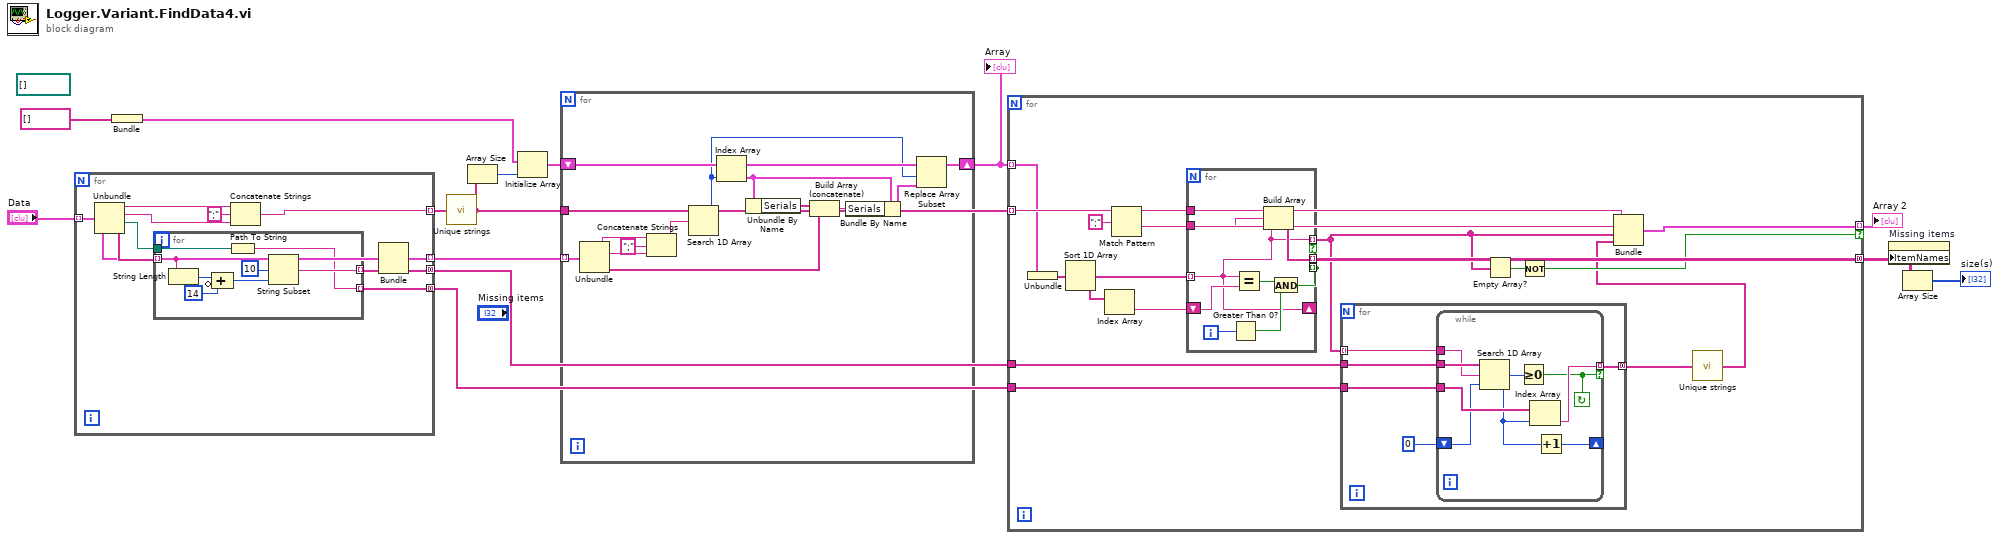
[diagram p0: block diagram]
diagram:
  (unwired) path[] [] ("Serials")
  n1 = for {
    tunnel: "Data" -> [w21] mode=indexing
    tunnel: [w18] -> w14 mode=indexing
    tunnel: [w20] -> w8 mode=indexing
    tunnel: [w16] -> w1 mode=concatenating
    tunnel: [w15] -> w2 mode=concatenating
    n2 = Unbundle(w21) -> ("Product"=w24:string, "Plate"=w23:string, "Path"=w17:path, "Serials"=w22:string[])
    n3 = for {
      tunnel: w22 -> [w31] mode=indexing
      tunnel: [w27] -> w15 mode=indexing
      tunnel: w17 -> [w26]
      tunnel: [w25] -> w16 mode=indexing
      n4 = String Length(string=w31) -> (length=w30:i32)
      n5 = Compound Arithmetic op=ADD(w30, invert 14 ("value")) -> (w28:i32)
      n6 = Path To String(path=w26) -> (string=w25:string)
      n7 = String Subset(string=w31, offset (0)=10 ("length (rest)"), length (rest)=w28) -> (substring=w27:string)
    }
    n8 = Concatenate Strings(w24, ";" ("string"), w23) -> (w18:string)
    n9 = Bundle(cluster=w21, "Serials"=w15) -> (w20:T3)  [unwired: 3 in]
  }
  n10 = Bundle("Serials"=string[] []) -> (w10:cluster{"Serials":string[]})  [unwired: 1 in]
  n11 = call "Unique strings.vi"("values in"=w14) -> ("unique values"=w6:string[])
  n12 = Array Size(array=w6) -> (size(s)=w12:i32)
  n13 = Initialize Array(w10, w12) -> (w9:cluster{"Serials":string[]}[])
  n14 = for {
    tunnel: w6 -> [w43]
    tunnel: w8 -> [w46] mode=indexing
    shift-right: [w41] -> w7
    shift-left: w9 -> [w40]
    n15 = Unbundle(w46) -> ("Product"=w45:string, "Plate"=w44:string, "Serials"=w35:string[])  [unwired: 1 out]
    n16 = Concatenate Strings(w45, ";" ("string"), w44) -> (w42:string)
    n17 = Search 1D Array(1D array=w43, element=w42) -> (index of element=w39:i32)  [unwired: 1 in]
    n18 = Index Array(array=w40, index=w39) -> (element=w37:cluster{"Serials":string[]})
    n19 = Unbundle By Name(w37) -> ("Serials"=w36:string[])
    n20 = Build Array (concatenate)(w36, w35) -> (w34:string[])
    n21 = Bundle By Name(cluster=w37, "Serials"=w34) -> (w38:cluster{"Serials":string[]})
    n22 = Replace Array Subset(array=w40, new element=w38, index=w39) -> (w41:cluster{"Serials":string[]}[])
  }
  "Array" <- w7
  n23 = for {
    tunnel: w7 -> [w59] mode=indexing
    tunnel: w6 -> [w61] mode=indexing
    tunnel: [w58] -> w4 mode=concatenating
    tunnel: [w54] -> w5 mode=indexing if=w53
    tunnel: w2 -> [w51]
    tunnel: w1 -> [w50]
    n24 = Unbundle(w59) -> ("Serials"=w63:string[])
    n25 = Sort 1D Array(array=w63) -> (sorted array=w52:string[])
    n26 = Index Array(array=w52) -> (element=w62:string)  [unwired: 1 in]
    n27 = Match Pattern(string=w61, regular expression=";") -> (before substring=w56:string, after substring=w55:string)  [unwired: 1 in, 2 out]
    n28 = for {
      shift-right: [w78] -> _
      shift-left: w62 -> [w84]
      tunnel: w52 -> [w78] mode=indexing
      tunnel: [w79] -> w58 mode=indexing if=w77
      tunnel: w56 -> [w81]
      tunnel: w55 -> [w80]
      tunnel: [w77] -> _ mode=indexing
      tunnel: [w78] -> w47 mode=indexing if=w77
      i -> [w85]
      n29 = Greater Than 0?(x=w85) -> (x > 0?=w82:bool)
      n30 = Equal?(x=w78, y=w84) -> (x = y?=w83:bool)
      n31 = Build Array(w81, w80, w78) -> (w79:string[])
      n32 = Compound Arithmetic op=AND(w83, w82) -> (w77:bool)
    }
    n33 = for {
      tunnel: w51 -> [w68]
      tunnel: w50 -> [w66]
      tunnel: w47 -> [w67] mode=indexing
      tunnel: [w64] -> w49 mode=concatenating
      n34 = while {
        tunnel: w68 -> [w76]
        tunnel: w67 -> [w75]
        tunnel: w66 -> [w74]
        shift-right: [w71] -> _
        shift-left: 0 -> [w73]
        tunnel: [w70] -> w64 mode=indexing if=w69
        stop <- w69 continue-if-true
        n35 = Search 1D Array(1D array=w76, element=w75, start index (0)=w73) -> (index of element=w72:i32)
        n36 = Greater Or Equal To 0?(x=w72) -> (x >= 0?=w69:bool)
        n37 = Index Array(array=w74, index=w72) -> (element=w70:string)
        n38 = Increment(x=w72) -> (x+1=w71:i32)
      }
    }
    n39 = Empty Array?(array=w47) -> (empty?=w57:bool)
    n40 = Not(x=w57) -> (.not. x?=w53:bool)
    n41 = call "Unique strings.vi"("values in"=w49) -> ("unique values"=w48:string[])
    n42 = Bundle("value"=w56, "value"=w55, w47, "unique values"=w48) -> (w54:T4)  [unwired: 1 in]
  }
  "Array 2" <- w5
  n43 = property on="Missing items" class="MCListbox (strict)"("ItemNames"=w4) -> ()  [unwired: 2 in, 2 out]
  n44 = Array Size(array=w4) -> (size(s)=→"size(s)":i32[])
